vi "Group_Cluster.vi"() -> ()   [LabVIEW 2014]
uses:
  <vilib>/Utility/file.llb/Read From Spreadsheet File (DBL).vi
  <vilib>/Utility/file.llb/Read From Spreadsheet File (I64).vi
panel:
  in  "Clustering":path
  in  "Cluster_Number":i32
  out "Inverse_W_grouped":dbl[][](array[numeric])
  out "N(number of Clusters)":i32
  in  "Inverse_W.txt":path
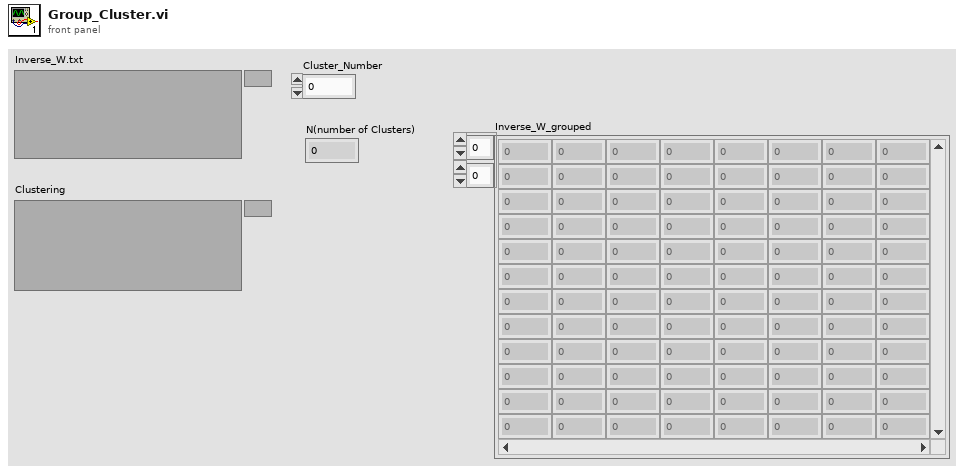
[diagram p1: front panel]
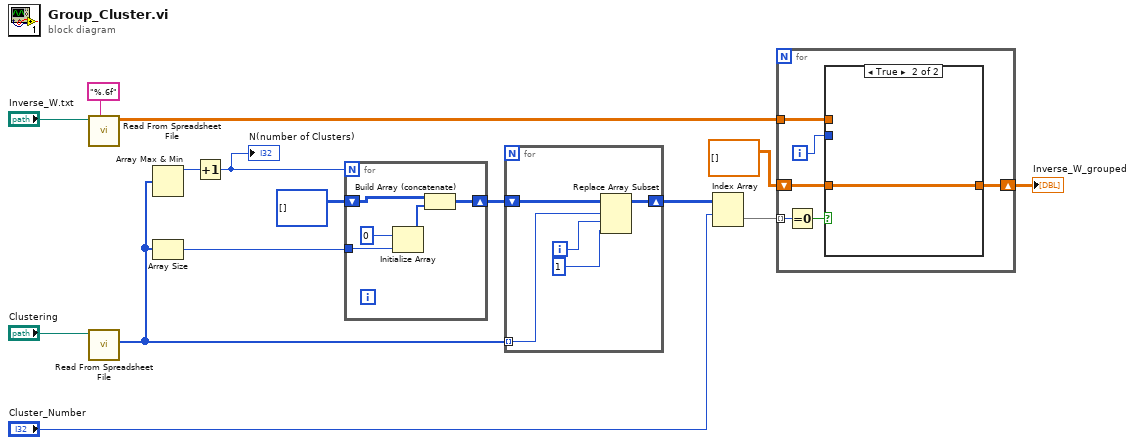
[diagram p0: block diagram]
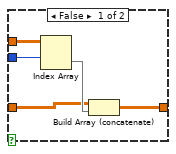
[diagram p2: hidden frame]
diagram:
  n1 = call-poly <vilib>:"Read From Spreadsheet File.vi"("format (%.3f)"="%.6f", "file path (dialog if empty)"="Inverse_W.txt") -> ("all rows"=w7:dbl[][])  [unwired: 5 in, 4 out]
  n2 = call-poly <vilib>:"Read From Spreadsheet File.vi"("file path (dialog if empty)"="Clustering") -> ("first row"=w1:i64[])  [unwired: 6 in, 4 out]
  n3 = Array Max & Min(array=w1) -> (max value=w13:i64)  [unwired: 3 out]
  n4 = Array Size(array=w1) -> (size(s)=w12:i32)
  n5 = Increment(x=w13) -> (x+1=w9:i64)
  "N(number of Clusters)" <- w9
  n6 = for {
    N: w9 -> [_]
    tunnel: w12 -> [w16]
    shift-right: [w19] -> w10
    shift-left: i32[][] [] -> [w18]
    n7 = Initialize Array(0 ("dimension size"), w16) -> (w20:i32[])
    n8 = Build Array (concatenate)(w18, w20) -> (w19:i32[][])
  }
  n9 = for {
    shift-right: [w21] -> w8
    shift-left: w10 -> [w25]
    tunnel: w1 -> [w24] mode=indexing
    i -> [w23]
    n10 = Replace Array Subset(array=w25, new element=1 ("new element/subarray"), index (row)=w24, index (col)=w23) -> (w21:i32[][])
  }
  n11 = Index Array(array=w8, index (row)="Cluster_Number") -> (element=w6:i32[])  [unwired: 1 in]
  n12 = for {
    tunnel: w6 -> [w31] mode=indexing
    tunnel: w7 -> [w29]
    shift-right: [w27] -> w4
    shift-left: dbl[][] [] -> [w26]
    i -> [w28]
    n13 = Equal To 0?(x=w31) -> (x = 0?=w30:bool)
    n14 = case shown="True" w30 {
      tunnel: w29 -> [w36 _]
      tunnel: w28 -> [w35 _]
      tunnel: [w33 w37] -> w27
      tunnel: w26 -> [w32 w37]
      frame False {
        n15 = Index Array(array=w36, index (row)=w35) -> (element=w34:dbl[])  [unwired: 1 in]
        n16 = Build Array (concatenate)(w32, w34) -> (w33:dbl[][])
      }
      frame True {
      }
    }
  }
  "Inverse_W_grouped" <- w4
